vi "Furnace 1 PV.vi"(8 "error in":errorcluster) -> (0 "error out":errorcluster, 2 "Array":u8[](array[numeric]))   [LabVIEW 2014]
uses:
  <vilib>/rvi/eio/common/nirviEmuTemplateMethod_errors.vi
  <vilib>/eio/EIOMethodNode/EIOMethodNode.xnode
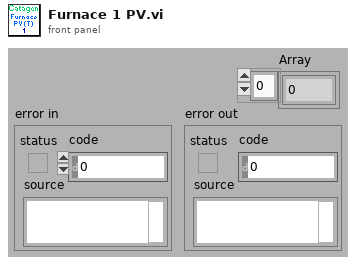
[diagram p1: front panel]
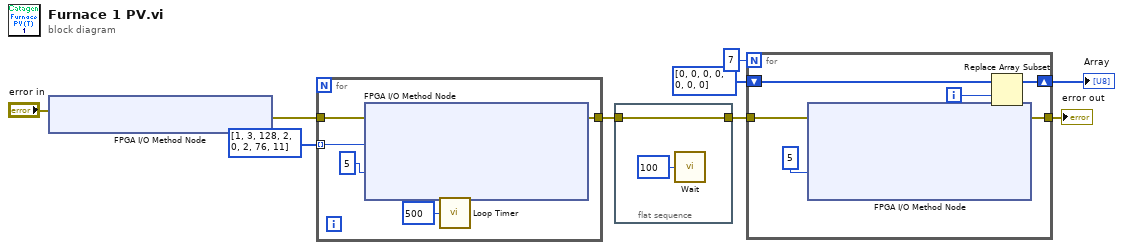
[diagram p0: block diagram]
diagram:
  n1 = xnode "FPGA I/O Method Node"("error in"="error in") -> ("error out"=w5:errorcluster)  [unwired: 1 in, 1 out]
  n2 = for {
    tunnel: u8[] [1, 3, 128, 2, 0, 2, 76, 11] -> [w13] mode=indexing
    tunnel: [w12] -> w4
    tunnel: w5 -> [w10]
    n3 = xnode "FPGA I/O Method Node"("error in"=w10, "Data"=w13, "Timeout (ms)"=5) -> ("error out"=w12:errorcluster)  [unwired: 1 in, 2 out]
    n4 = call "Loop Timer"("Count(uSec)"=u32 500 ("Count(mSec)")) -> ()  [unwired: 1 out]
  }
  n5 = flat-sequence {
    tunnel: w4 -> [w16]
    tunnel: [w16] -> w3
    frame #0 {
      n6 = call "Wait"("Count(mSec)"=u32 100) -> ()  [unwired: 1 out]
    }
  }
  n7 = for {
    N: 7 -> [_]
    tunnel: w3 -> [w23]
    shift-right: [w19] -> w6
    shift-left: u8[] [0, 0, 0, 0, 0, 0, 0] -> [w21]
    tunnel: [w17] -> w1
    i -> [w18]
    n8 = xnode "FPGA I/O Method Node"("error in"=w23, "Timeout (ms)"=5) -> ("error out"=w17:errorcluster, "Data"=w20:u8)  [unwired: 1 in, 2 out]
    n9 = Replace Array Subset(array=w21, new element=w20, index=w18) -> (w19:u8[])
  }
  "Array" <- w6
  "error out" <- w1
